vi "close.vi"(8 "error in":errorcluster, 11 "EthernetIP runtime in":refnum<class "EIP Tags Runtime.lvclass">) -> (0 "error out":errorcluster)   [LabVIEW 2013, in "EIP Tags Runtime.lvclass"]
doc: "Provides an interface for terminating a module instance. While this interface performs no operations, a child should close and deallocate any open references or memory."
uses:
  EIP Tags Runtime.lvclass
  EIP Tags Runtime.lvclass/EIP Tags Runtime.ctl
  <vilib>/ethernetip/ethernetip.lvlib
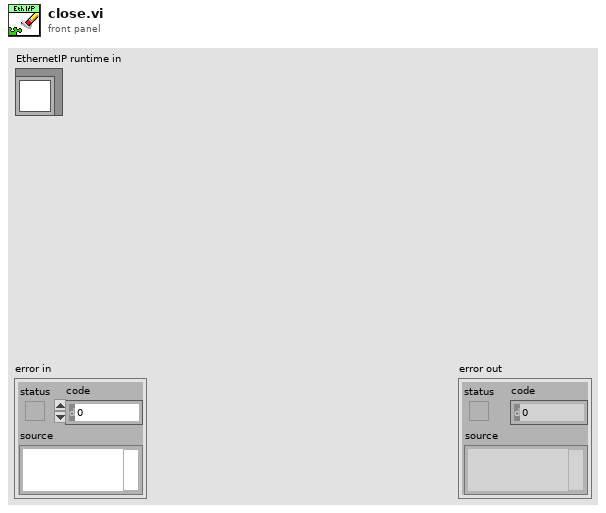
[diagram p1: front panel]
types:
  T1 = typedef "ethernetip.lvlib/ethernetip.ctl" = refnum<k21>
  T2 = typedef "EIP Tags Runtime.lvclass/assembly data spec.ctl" = cluster{"Instance ID":u32, "specification":T3[], "big endian?":bool}
  T3 = typedef "EIP Tags Runtime.lvclass/conversion specification.ctl" = cluster{"data type":T4, "data index":i32, "byte index":i32, "subindex":i32}
  T4 = typedef "tag bus.lvlib/tag descriptor.lvclass/Data Type.ctl" = enum16{"Double", "Single", "I64", "I32", "I16", "I8", "U64", "U32", "U16", "U8", "Boolean", "String", "Array of Double", "Array of Single", "Array of I64", "Array of I32", "Array of I16", "Array of I8", "Array of U64", "Array of U32", "Array of U16", "Array of U8", "Array of Boolean", "Array of String"}
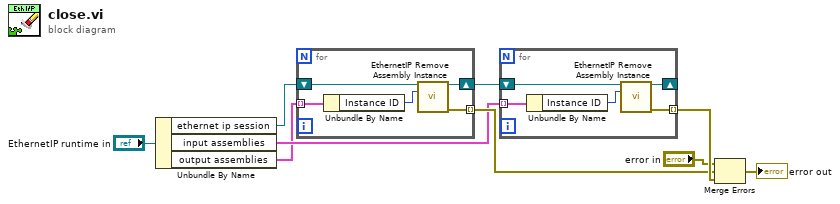
[diagram p0: block diagram]
diagram:
  n1 = Unbundle By Name("EthernetIP runtime in") -> ("ethernet ip session"=w4:T1, "input assemblies"=w2:T2[], "output assemblies"=w1:T2[])
  n2 = for {
    tunnel: [w14] -> w7 mode=indexing
    shift-right: [w12] -> w3
    shift-left: w4 -> [w13]
    tunnel: w1 -> [w11] mode=indexing
    n3 = Unbundle By Name(w11) -> ("Instance ID"=w10:u32)
    n4 = call <vilib>:"EthernetIP Remove Assembly Instance.vi"("Session in"=w13, "Instance ID"=w10) -> ("Session out"=w12:T1, "error out"=w14:errorcluster)  [unwired: 12 in]
  }
  n5 = for {
    tunnel: [w19] -> w8 mode=indexing
    shift-right: [w17] -> _
    shift-left: w3 -> [w18]
    tunnel: w2 -> [w16] mode=indexing
    n6 = Unbundle By Name(w16) -> ("Instance ID"=w15:u32)
    n7 = call <vilib>:"EthernetIP Remove Assembly Instance.vi"("Session in"=w18, "Instance ID"=w15) -> ("Session out"=w17:T1, "error out"=w19:errorcluster)  [unwired: 12 in]
  }
  n8 = Merge Errors("error in", w7, w8) -> (→"error out":errorcluster)
